vi "Send.vi"(0 "STOMP in":refnum<class "STOMP.lvclass">, 1 "Destination":string, 2 "Body":string, 3 "headers":T1[](array[typedef]), 5 "error in (no error)":errorcluster, 6 "Receipt?":bool) -> (14 "STOMP out":refnum<class "STOMP.lvclass">, 19 "error out":errorcluster)   [LabVIEW 2017, in "STOMP.lvclass"]
uses:
  STOMP.lvclass
  Typedefs/Type_FrameHeader.ctl
  Typedefs/Type_ClientFrame.ctl
  Typedefs/Type_ClientFrameType.ctl
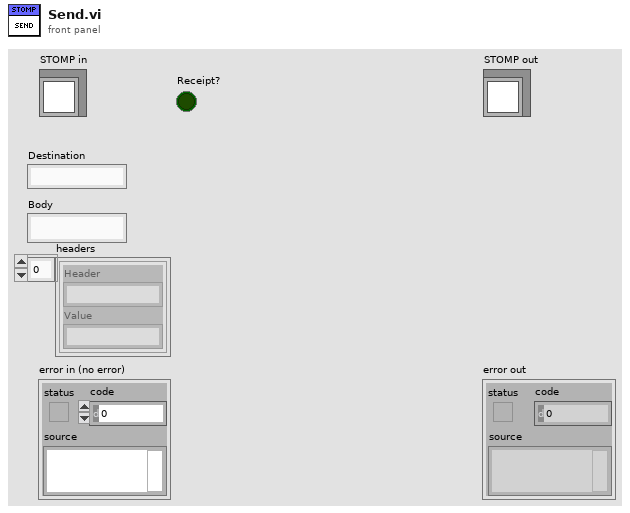
[diagram p1: front panel]
types:
  T1 = typedef "STOMP.lvclass/Type_FrameHeader.ctl" = cluster{"Header":string, "Value":string}
  T2 = typedef "STOMP.lvclass/Type_ClientFrameType.ctl" = enum16{"Undefined", "SEND", "SUBSCRIBE", "UNSUBSCRIBE", "BEGIN", "COMMIT", "ABORT", "ACK", "NACK", "DISCONNECT"}
  T3 = typedef "STOMP.lvclass/Type_ClientFrame.ctl" = cluster{"Type":T2, "Headers":T1[], "Body":string}
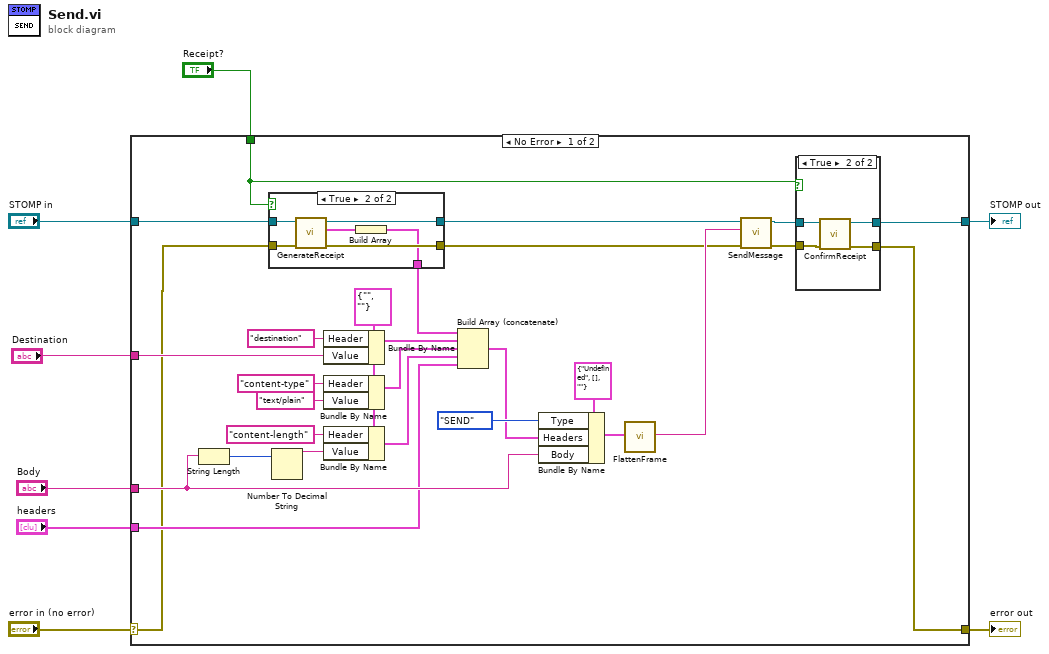
[diagram p0: block diagram]
diagram:
  n1 = case shown="No Error" "error in (no error)" {
    selector: "error in (no error)" -> [w19 w52]
    tunnel: [w13 w52] -> w7
    tunnel: [w12 w51] -> w5
    tunnel: "STOMP in" -> [w20 w51]
    tunnel: "Destination" -> [w34 _]
    tunnel: "Body" -> [w26 _]
    tunnel: "headers" -> [w22 _]
    tunnel: "Receipt?" -> [w11 _]
    frame No Error {
      w21 = T1 {"Header"="", "Value"=""}
      n2 = String Length(string=w26) -> (length=w10:i32)
      n3 = case shown="True" w11 {
        tunnel: w20 -> [w44 w50]
        tunnel: w19 -> [w43 w49]
        tunnel: [w44 w48] -> w18
        tunnel: [w43 w47] -> w17
        tunnel: [_ w45] -> w16
        frame False {
        }
        frame True {
          n4 = call-dynamic "GenerateReceipt.vi"("error in (no error)"=w49, "STOMP in"=w50) -> ("error out"=w47:errorcluster, "Receipt Header"=w46:T1, "STOMP out"=w48:refnum<class "STOMP.lvclass">)  [unwired: 7 in]
          n5 = Build Array(w46) -> (w45:T1[])
        }
      }
      n6 = Number To Decimal String(number=w10) -> (decimal integer string=w25:string)  [unwired: 1 in]
      n7 = Bundle By Name(cluster=w21, "Header"="destination", "Value"=w34) -> (w30:T1)
      n8 = Bundle By Name(cluster=w21, "Header"="content-type", "Value"="text/plain") -> (w29:T1)
      n9 = Bundle By Name(cluster=w21, "Header"="content-length", "Value"=w25) -> (w9:T1)
      n10 = Build Array (concatenate)(w16, w30, w29, w9, w22) -> (w28:T1[])
      n11 = Bundle By Name(cluster=T3 {"Type"=enum."Undefined", "Headers"=[], "Body"=""} ("Type_ClientFrame"), "Type"=Type_ClientFrameType."SEND", "Headers"=w28, "Body"=w26) -> (w24:T3)
      n12 = call "FlattenFrame.vi"("Client Frame"=w24) -> ("flattened frame"=w23:string)  [unwired: 18 in]
      n13 = call-dynamic "SendMessage.vi"("error in (no error)"=w17, "data in"=w23, "STOMP in"=w18) -> ("error out"=w14:errorcluster, "STOMP out"=w15:refnum<class "STOMP.lvclass">)  [unwired: 7 in]
      n14 = case shown="True" w11 {
        tunnel: w15 -> [w37 w42]
        tunnel: w14 -> [w38 w41]
        tunnel: [w38 w40] -> w13
        tunnel: [w37 w39] -> w12
        frame False {
        }
        frame True {
          n15 = call-dynamic "ConfirmReceipt.vi"("error in (no error)"=w41, "STOMP in"=w42) -> ("error out"=w40:errorcluster, "STOMP out"=w39:refnum<class "STOMP.lvclass">)  [unwired: 8 in]
        }
      }
    }
    frame Error {
    }
  }
  "error out" <- w7
  "STOMP out" <- w5
